vi "Autotest_Instr.vi"(8 "error in (no error)":errorcluster caption="entrée d'erreur (pas d'erreur)", 11 "Class Instrument Firebase en entrée":refnum<class "Class Instrument Firebase Altyor.lvclass">) -> (0 "error out":errorcluster caption="sortie d'erreur", 3 "Class Instrument Firebase en sortie":refnum<class "Class Instrument Firebase Altyor.lvclass">)   [LabVIEW 2020, in "Library Instrument & Equipement.lvlib" / "Library Instruments.lvlib" / "Class Instrument Firebase Altyor.lvclass"]
uses:
  Class Instrument Firebase Altyor.lvclass
  C:/Users/ngarcin/OneDrive - Altyor/Standard TB/Class/Instrument/Instrument (Default)/Class Instrument (Default).lvclass
  Class Instrument Firebase Altyor.lvclass/Class Instrument Firebase Altyor.ctl
  Firebase/Source/Firebase Altyor/Firebase Altyor.lvclass
  C:/Users/ngarcin/OneDrive - Altyor/Standard TB/Class/Firebase/Source/Firebase Driver/Firebase Driver.lvclass
  Instrument (Default)/Class Instrument (Default).lvclass
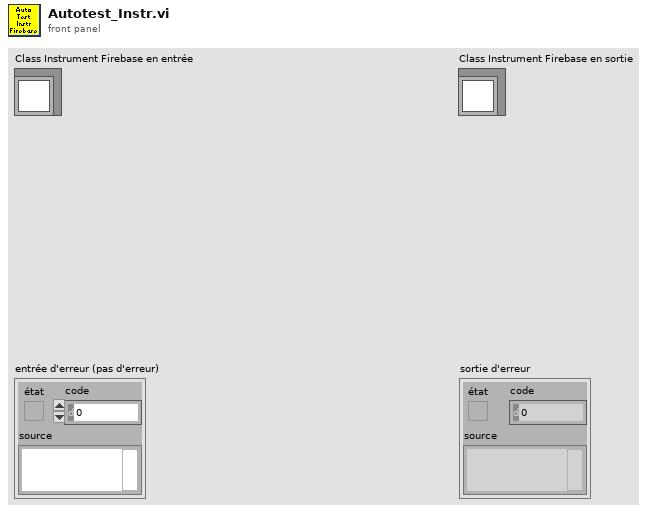
[diagram p1: front panel]
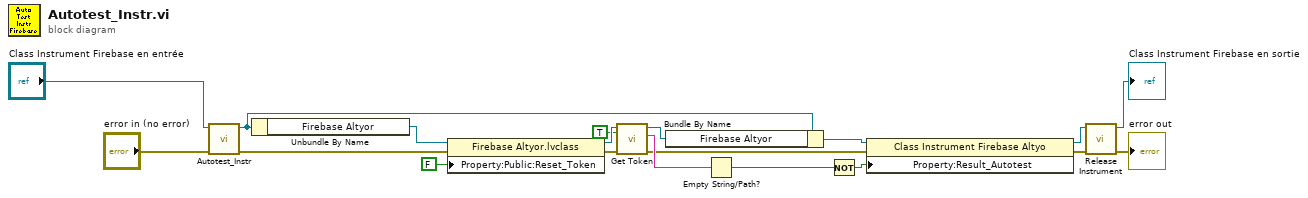
[diagram p0: block diagram]
diagram:
  n1 = call-parent "Autotest_Instr.vi"("error in (no error)"="error in (no error)", "Class Instrument (Default) en entrée"="Class Instrument Firebase en entrée") -> ("error out"=w17:errorcluster, "Class Instrument (Default) en sortie"=w7:refnum<class "Class Instrument Firebase Altyor.lvclass">)  [unwired: 8 in]
  n2 = Unbundle By Name(w7) -> ("Firebase Altyor"=w10:refnum<class "Firebase Altyor.lvclass">)
  n3 = property class="Firebase Altyor.lvclass"(reference=w10, error in=w17, "Property:Public:Reset_Token"=FALSE ("Reset_Token")) -> (reference out=w14:refnum<class "Firebase Altyor.lvclass">, error out=w15:errorcluster)
  n4 = call-dynamic "Get Token.vi"("error in (no error)"=w15, "Reset"=TRUE, "Build Library FireBase.lvlib:Firebase (Default) IN"=w14) -> ("error out"=w6:errorcluster, "idToken"=w13:string, "Build Library FireBase.lvlib:Firebase (Default) Out"=w11:refnum<class "Firebase Altyor.lvclass">)  [unwired: 6 in]
  n5 = Bundle By Name(cluster=w7, "Firebase Altyor"=w11) -> (w4:refnum<class "Class Instrument Firebase Altyor.lvclass">)
  n6 = Empty String/Path?(string/path=w13) -> (empty?=w12:bool)
  n7 = Not(x=w12) -> (.not. x?=w2:bool)
  n8 = property class="Class Instrument Firebase Altyo"(reference=w4, error in=w6, "Property:Result_Autotest"=w2) -> (reference out=w3:refnum<class "Class Instrument Firebase Altyor.lvclass">, error out=w5:errorcluster)
  n9 = call-dynamic "Release Instrument.vi"("error in (no error)"=w5, "Class Instrument (Default) en entrée"=w3) -> ("error out"=→"error out":errorcluster, "Class Instrument (Default) en sortie"=→"Class Instrument Firebase en sortie":refnum<class "Class Instrument Firebase Altyor.lvclass">)  [unwired: 8 in]
